vi "InspectCall.vi"(6 "Error":errorcluster, 7 "Actor":refnum<class "Actor.lvclass">, 11 "Message":refnum<class "Msg.lvclass">) -> (2 "Call":bool=TRUE, 3 "Message":refnum<class "Msg.lvclass">, 4 "Error":errorcluster, 5 "Actor":refnum<class "Actor.lvclass">)   [LabVIEW 2020, in "_Template.lvlib" / "{{Actor}}.lvlib" / "Actor.lvclass"]
uses:
  Actor.lvclass
  Actor.lvclass/Actor.ctl
  jettl/jettl/Actor/Actor.lvclass
  jettl/jettl/Msg/Msg.lvclass
panel:
  # "This front panel should not be manipulated."
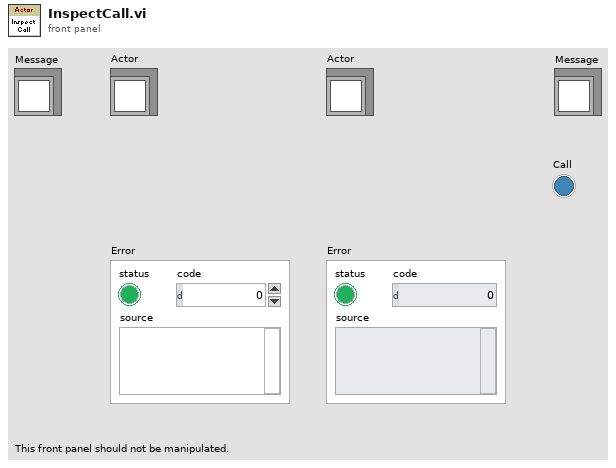
[diagram p1: front panel]
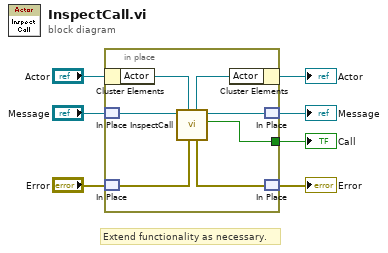
[diagram p0: block diagram]
diagram:
  # "Extend functionality as necessary."
  n1 = in-place {
    in-place-border: [w8] -> w1
    n2 = in-place-cluster #1("Actor") -> ("Actor"=w14:refnum<class "Actor.lvclass">)
    n3 = in-place-match #2("Message") -> (w11:refnum<class "Msg.lvclass">)
    n4 = in-place-match #3("Error") -> (w10:errorcluster)
    n5 = call-dynamic "InspectCall.vi"("Error"=w10, "Actor"=w14, "Message"=w11) -> ("Call"=w8:bool, "Message"=w12:refnum<class "Msg.lvclass">, "Error"=w9:errorcluster, "Actor"=w13:refnum<class "Actor.lvclass">)  [unwired: 5 in]
    n6 = in-place-cluster #1("Actor"=w13) -> (→"Actor":refnum<class "Actor.lvclass">)
    n7 = in-place-match #2(w12) -> (→"Message":refnum<class "Msg.lvclass">)
    n8 = in-place-match #3(w9) -> (→"Error":errorcluster)
  }
  "Call" <- w1
